vi "test VIT Verify g-cli.vi"(8 "error in":errorcluster, 11 "Testing Approval Tests in":refnum<class "VITester Extension Tests.lvclass">) -> (0 "error out":errorcluster, 3 "Testing Approval Tests out":refnum<class "VITester Extension Tests.lvclass">)   [LabVIEW 2026, in "VITester Extension Tests.lvclass"]
uses:
  VITester Extension Tests.lvclass
  VITester Extension Tests.lvclass/VITester Extension Tests.ctl
  Source/Extensions/VITester.Extension/VITester.Extension.lvlib
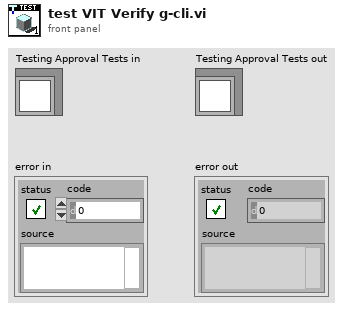
[diagram p1: front panel]
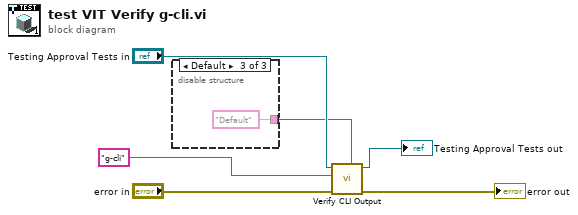
[diagram p0: block diagram]
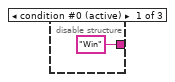
[diagram p2: hidden frame]
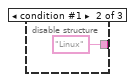
[diagram p3: hidden frame]
diagram:
  n1 = disable-structure shown="Default" {
    disable-tunnel: ["Win" ("Label") "Linux" ("Label") "Default" ("Label")] -> w1
    frame condition #0 (active) {
    }
    frame condition #1 {
    }
    frame condition #2 {
    }
  }
  n2 = call "Verify CLI Output.vi"("Label"=w1, "error in"="error in", "command line"="g-cli", "TestCase in"="Testing Approval Tests in") -> ("error out"=→"error out":errorcluster, "TestCase out"=→"Testing Approval Tests out":refnum<class "VITester Extension Tests.lvclass">)  [unwired: 6 in]
